vi "写入Color.vi"(8 "error in (no error)":errorcluster caption="错误输入（无错误）", 10 "Color":string, 11 "animal输入":refnum<class "animal.lvclass">) -> (0 "error out":errorcluster caption="错误输出", 3 "animal输出":refnum<class "animal.lvclass">)   [LabVIEW 2018, in "animal.lvclass"]
uses:
  animal.lvclass
  animal.lvclass/animal.ctl
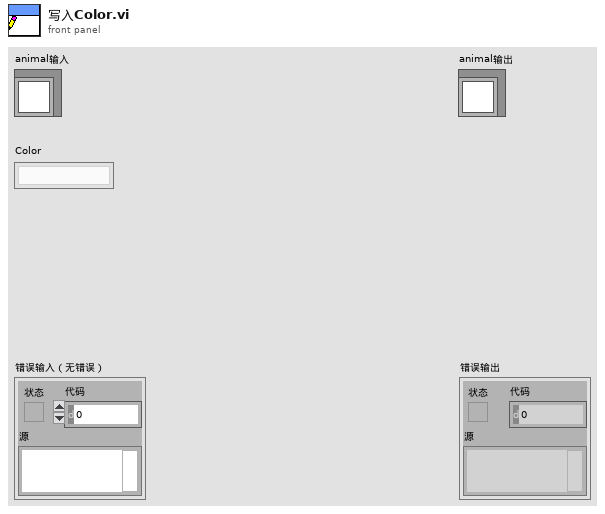
[diagram p1: front panel]
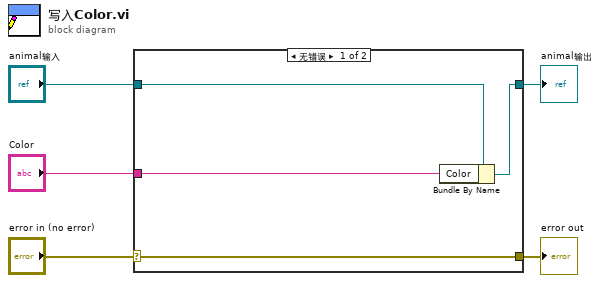
[diagram p0: block diagram]
diagram:
  n1 = case shown="无错误" "error in (no error)" {
    selector: "error in (no error)" -> [w9 w10]
    tunnel: [w9 w10] -> w4
    tunnel: [w7 w11] -> w2
    tunnel: "animal输入" -> [w8 w11]
    tunnel: "Color" -> [w6 _]
    frame No Error {
      n2 = Bundle By Name(cluster=w8, "Color"=w6) -> (w7:refnum<class "animal.lvclass">)
    }
    frame Error {
    }
  }
  "error out" <- w4
  "animal输出" <- w2
